vi "UE9 DAC Dual Function Generator.vi"() -> ()   [LabVIEW 2021]
uses:
  <vilib>/measure/NI_MABase.lvlib
panel:
  in  "Function 1":u16(ring) items=["Sine Wave", "Triangle Wave", "Square Wave", "Sawtooth Wave"]
  in  "Min Voltage 1":dbl=0.5 min=0.0 max=5.0 step=0.1 format="%.2f"
  in  "Max Voltage 1":dbl=4.5 min=0.0 max=5.0 step=0.1 format="%.2f"
  in  "Frequency (Hz) 1":dbl=1.0 step=0.1 format="%.3f"
  in  "Update Interval (ms)":u32=20
  out "Error":string
  in  "Function 0":u16(ring) items=["Sine Wave", "Triangle Wave", "Square Wave", "Sawtooth Wave"]
  in  "Min Voltage 0":dbl=0.5 min=0.0 max=5.0 step=0.1 format="%.2f"
  in  "Max Voltage 0":dbl=4.5 min=0.0 max=5.0 step=0.1 format="%.2f"
  out "Waveform Chart":cluster{dbl, dbl}(graph)
  in  "Frequency 0 (Hz)":dbl=1.0 step=0.1 format="%.3f"
  in  "Stop":bool
  # "Updates DAC0 & DAC1 at the specified update interval in order to build time series waveforms.  The\nupdate interval is set to 20 ms by default, but can be set lower based on the execution times\ndiscussed in Section 3.1 of the UE9 User's Guide.  Uses the first found USB UE9.\n\nWith a software timed application such as this, you might be able to reduce timing jitter (caused\nby the operating system) by increasing the priority of this process (labview.exe) in Windows\nTask Manager."
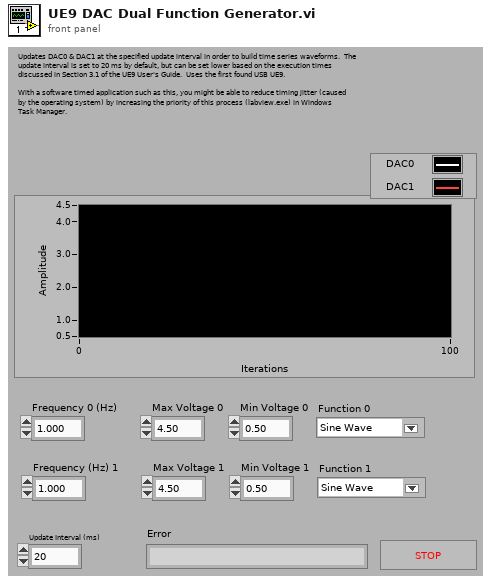
[diagram p1: front panel]
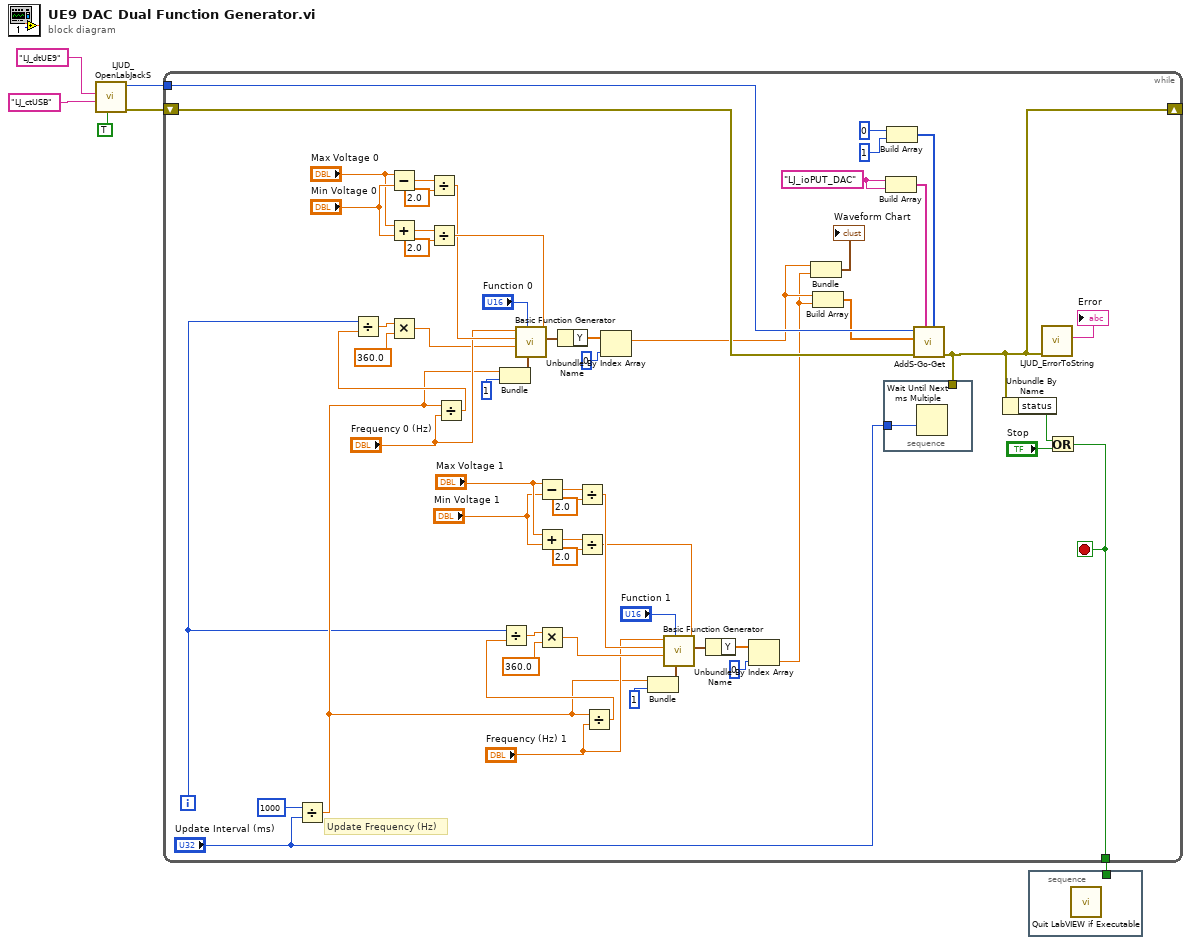
[diagram p0: block diagram]
diagram:
  n1 = call "LJUD_OpenLabJackS.vi"("FirstFound"=TRUE, "ConnectionType"="LJ_ctUSB", "DeviceType"="LJ_dtUE9") -> ("error out"=w2:errorcluster, "Handle"=w1:i32)  [unwired: 6 in, 1 out]
  n2 = while {
    tunnel: w1 -> [w32]
    shift-left: w2 -> [w33]
    shift-right: [w34] -> _
    tunnel: [w42] -> w6
    i -> [w11]
    stop <- w42 stop-if-true
    w35 = "LJ_ioPUT_DAC" ("IOType")
    # "Update Frequency (Hz)"
    n3 = Divide(x=u32 1000, y="Update Interval (ms)") -> (x/y=w12:dbl)
    n4 = Subtract(x="Max Voltage 0", y="Min Voltage 0") -> (x-y=w62:dbl)
    n5 = Add(x="Max Voltage 0", y="Min Voltage 0") -> (x+y=w59:dbl)
    n6 = Divide(x=w62, y=2.0) -> (x/y=w54:dbl)
    n7 = Divide(x=w59, y=2.0) -> (x/y=w55:dbl)
    n8 = Divide(x=w12, y="Frequency 0 (Hz)") -> (x/y=w64:dbl)
    n9 = Divide(x=w11, y=w64) -> (x/y=w63:dbl)
    n10 = Multiply(x=w63, y=360.0) -> (x*y=w51:dbl)
    n11 = Bundle(w12, 1) -> (w49:cluster{dbl, i32})  [unwired: 1 in]
    n12 = call <vilib>:"Basic Function Generator.vi"("offset"=w55, "sampling info"=w49, "signal type"="Function 0", "phase"=w51, "amplitude"=w54, "frequency"="Frequency 0 (Hz)") -> ("signal out"=w48:waveform(dbl))  [unwired: 3 in, 2 out]
    n13 = Subtract(x="Max Voltage 1", y="Min Voltage 1") -> (x-y=w19:dbl)
    n14 = Add(x="Max Voltage 1", y="Min Voltage 1") -> (x+y=w22:dbl)
    n15 = Unbundle By Name(w48) -> ("Y"=w47:dbl[])
    n16 = Divide(x=w19, y=2.0) -> (x/y=w24:dbl)
    n17 = Divide(x=w22, y=2.0) -> (x/y=w23:dbl)
    n18 = Divide(x=w12, y="Frequency (Hz) 1") -> (x/y=w17:dbl)
    n19 = Divide(x=w11, y=w17) -> (x/y=w18:dbl)
    n20 = Multiply(x=w18, y=360.0) -> (x*y=w26:dbl)
    n21 = Index Array(array=w47, index=0 ("Index")) -> (element=w9:dbl)
    n22 = Bundle(w12, 1) -> (w28:cluster{dbl, i32})  [unwired: 1 in]
    n23 = call <vilib>:"Basic Function Generator.vi"("offset"=w23, "sampling info"=w28, "signal type"="Function 1", "phase"=w26, "amplitude"=w24, "frequency"="Frequency (Hz) 1") -> ("signal out"=w29:waveform(dbl))  [unwired: 3 in, 2 out]
    n24 = Unbundle By Name(w29) -> ("Y"=w30:dbl[])
    n25 = Index Array(array=w30, index=0 ("Index")) -> (element=w8:dbl)
    n26 = Bundle(w9, w8) -> (→"Waveform Chart":cluster{dbl, dbl})  [unwired: 1 in]
    n27 = Build Array(w9, w8) -> (w10:dbl[])
    n28 = Build Array(w35, w35) -> (w36:string[])
    n29 = Build Array(0 ("Input Element"), 1 ("Input Element")) -> (w37:i32[])
    n30 = call "AddS-Go-Get.vi"("Channels"=w37, "IOTypes"=w36, "error in"=w33, "Values Write"=w10, "Handle In"=w32) -> ("error out"=w34:errorcluster)  [unwired: 4 in, 2 out]
    n31 = stacked-sequence {
      tunnel: "Update Interval (ms)" -> [w65]
      tunnel: w34 -> [_]
      frame #0 {
        n32 = Wait Until Next ms Multiple(millisecond multiple=w65) -> ()  [unwired: 1 out]
      }
    }
    n33 = Unbundle By Name(w34) -> ("status"=w43:bool)
    n34 = call "LJUD_ErrorToString.vi"("error in"=w34) -> ("String"=→"Error":string)  [unwired: 10 in]
    n35 = Or(x=w43, y="Stop") -> (x .or. y?=w42:bool)
  }
  n36 = stacked-sequence {
    tunnel: w6 -> [_]
    frame #0 {
      n37 = call "Quit LabVIEW if Executable.vi"() -> ()  [unwired: 1 in]
    }
  }
